vi "Extract Frame Structure.vi"(8 "Ring Refnum":refnum<vi>, 10 "MCListbox Refnum":refnum<vi>, 11 "Path in":refnum<vi>) -> (2 "array":string[][](array[string]))   [LabVIEW 2020]
panel:
  in  "Path":path
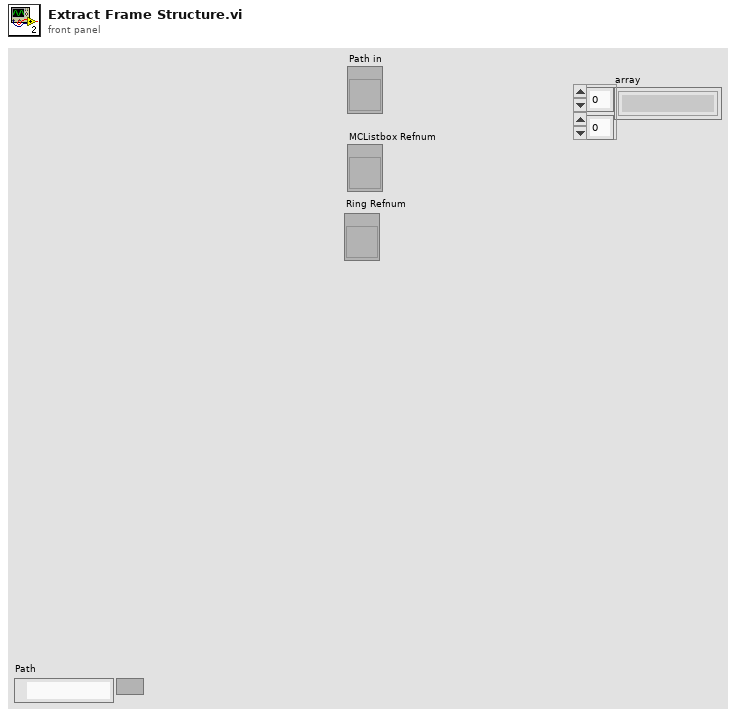
[diagram p1: front panel]
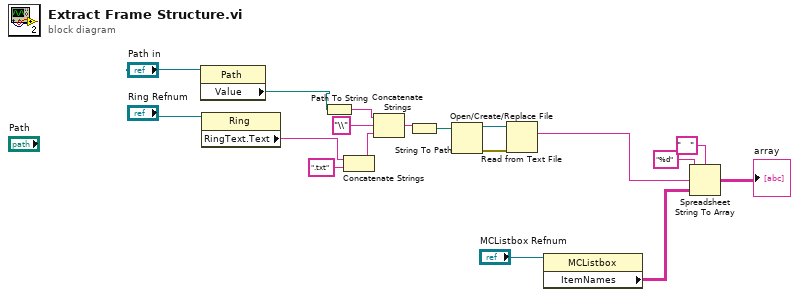
[diagram p0: block diagram]
diagram:
  n1 = property class="Path"(reference="Path in") -> ("Value"=w4:path)  [unwired: 1 in, 2 out]
  n2 = property on="Property Node" class="Ring"(reference="Ring Refnum") -> ("RingText.Text"=w12:string)  [unwired: 1 in, 2 out]
  n3 = Path To String(path=w4) -> (string=w16:string)
  n4 = Concatenate Strings(w12, ".txt" ("string")) -> (w10:string)
  n5 = Concatenate Strings(w16, "\\" ("string"), w10) -> (w14:string)
  n6 = String To Path(string=w14) -> (path=w13:path)
  n7 = Open/Create/Replace File(file path (use dialog)=w13) -> (refnum out=w3:refnum<file>, error out=w2:errorcluster)  [unwired: 5 in, 1 out]
  n8 = Read from Text File(file (use dialog)=w3, error in=w2) -> (text=w9:string)  [unwired: 2 in, 3 out]
  n9 = property on="Property Node" class="MCListbox"(reference="MCListbox Refnum") -> ("ItemNames"=w6:string[][])  [unwired: 1 in, 2 out]
  n10 = Spreadsheet String To Array(delimiter (Tab)="   ", format string="%d", spreadsheet string=w9, array type (2D Dbl)=w6) -> (array=→"array":string[][])
